vi "ArrayFloatToString.vi"(10 "2D Data":dbl[][](array[numeric]), 11 "1D Data":dbl[](array[numeric])) -> (2 "Array":string[][](array[string]), 3 "Array":string[](array[string]))   [LabVIEW 2020]
doc: "Convert float data to string data"
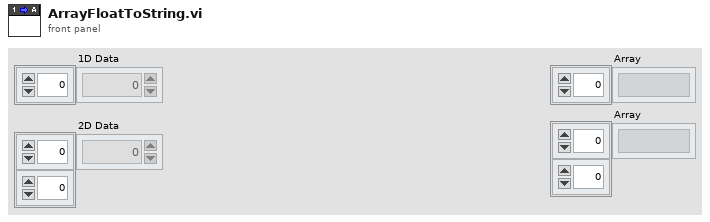
[diagram p1: front panel]
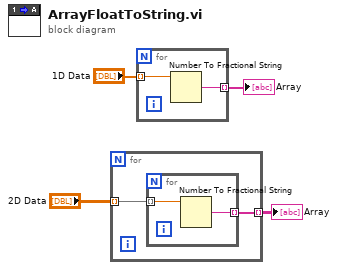
[diagram p0: block diagram]
diagram:
  n1 = for {
    tunnel: "2D Data" -> [w6] mode=indexing
    tunnel: [w5] -> w1 mode=indexing
    n2 = for {
      tunnel: w6 -> [w8] mode=indexing
      tunnel: [w7] -> w5 mode=indexing
      n3 = Number To Fractional String(number=w8) -> (F-format string=w7:string)  [unwired: 3 in]
    }
  }
  "Array" <- w1
  n4 = for {
    tunnel: "1D Data" -> [w10] mode=indexing
    tunnel: [w9] -> w3 mode=indexing
    n5 = Number To Fractional String(number=w10) -> (F-format string=w9:string)  [unwired: 3 in]
  }
  "Array" <- w3
